vi "sub_vi_write_final_file.vi"(6 "Extension":dbl, 8 "error in (no error)":errorcluster, 9 "1D data":string[](array[string]), 11 "Function":dbl) -> (0 "error out":errorcluster)   [LabVIEW 2016]
panel:
  out "Path":string
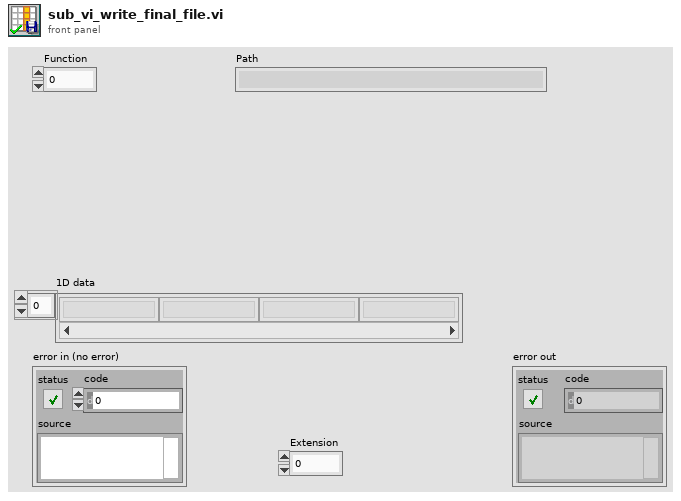
[diagram p1: front panel]
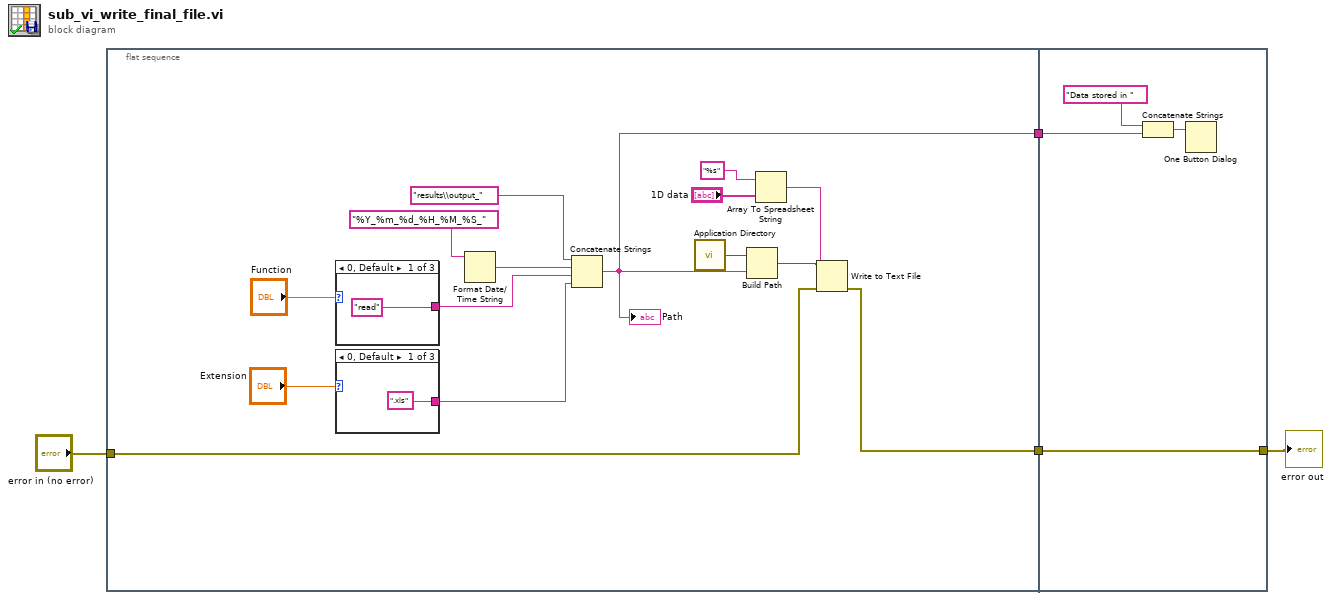
[diagram p0: block diagram]
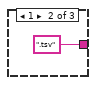
[diagram p2: hidden frame]
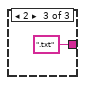
[diagram p3: hidden frame]
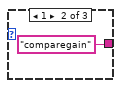
[diagram p4: hidden frame]
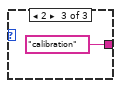
[diagram p5: hidden frame]
diagram:
  n1 = flat-sequence {
    tunnel: "error in (no error)" -> [w9]
    tunnel: [w8] -> w2
    tunnel: [w13] -> w1
    tunnel: [w29] -> w4
    tunnel: w2 -> [w29]
    tunnel: w1 -> [w27]
    frame #0 {
      n2 = case shown="0, Default" "Function" {
        tunnel: ["read" "comparegain" "calibration"] -> w14
        frame 0, Default {
        }
        frame 1 {
        }
        frame 2 {
        }
      }
      n3 = case shown="0, Default" "Extension" {
        tunnel: [".xls" ".tsv" ".txt"] -> w5
        frame 0, Default {
        }
        frame 1 {
        }
        frame 2 {
        }
      }
      n4 = Format Date/Time String(time format string (%c)="%Y_%m_%d_%H_%M_%S_") -> (date/time string=w15:string)  [unwired: 2 in]
      n5 = Concatenate Strings("results\\output_" ("string"), w15, w14, w5) -> (w13:string)
      "Path" <- w13
      n6 = call <vilib>:"Application Directory.vi"() -> ("Application Directory"=w19:path)
      n7 = Build Path(base path=w19, name or relative path=w13) -> (appended path=w10:path)
      n8 = Array To Spreadsheet String(array="1D data", 3:"%s" ("format string")) -> (spreadsheet string=w11:string)  [unwired: 1 in]
      n9 = Write to Text File(file (use dialog)=w10, text=w11, error in=w9) -> (error out=w8:errorcluster)  [unwired: 1 in, 2 out]
    }
    frame #1 {
      n10 = Concatenate Strings("Data stored in " ("string"), w27) -> (w26:string)
      n11 = One Button Dialog(message=w26) -> ()  [unwired: 1 in, 1 out]
    }
  }
  "error out" <- w4
